vi "State Machine.vi"() -> ()   [LabVIEW 2022 SP3]
uses:
  <vilib>/ErrorRing/Error Ring.xnode
  Control 9.ctl
panel:
  out "value voltage":dbl caption="Current Value (V)"
  out "Low Battery 4":bool caption="Low"
  out "timed out?\nSignal potentiometer":bool caption="Timeout"
  out "Low Battery 3":bool caption="Low"
  out "timed out?\nBattery potentiometer":bool caption="Timeout"
  in  "Knob 2":cluster{dbl, dbl}(knob)={0.0, 30.0} caption="Voltage Threshold" scale=0.0..12.0
  out "Low Battery 2":bool caption="Low"
  out "timed out?\nLink Quality\nThermometer":bool caption="Timeout"
  out "Low Battery":bool caption="Low"
  out "timed out?\nBattery Thermometer":bool caption="Timeout"
  out "Time Stamp 2":timestamp format="%<%d/%m/%y>T"
  out "Time Stamp":timestamp format="%<%H:%M>T"
  in  "Start/ pause":bool
  in  "Stop button":bool
  in  "Knob":cluster{dbl, dbl}(knob)={0.0, 30.0} caption="Temperature Threshold" scale=-20.0..60.0
  out "Meter":dbl(knob) caption="Voltage" scale=0.0..10.0
  out "Thermometer":dbl(slide) caption="Temperature" scale=0.0..100.0
  in  "Error In":errorcluster
  in  "Set lower voltage threshold":sgl=-1.0
  in  "Set upper voltage threshold":sgl=12.0
  out "Too High Voltage":bool
  in  "Set upper temperature threshold":sgl=30.0
  in  "Set lower temperature threshold":sgl=10.0
  out "Too hot":bool
  out "Too cold":bool
  out "min volt":sgl caption="Minimum (V)"
  out "max volt":sgl caption="Maximum (V)"
  out "mean volt":T1 caption="Mean (V)"
  out "min temp":sgl caption="Minimum (°C)"
  out "max temp":sgl caption="Maximum (°C)"
  out "mean temp":sgl caption="Mean (°C)"
  out "temperature":sgl(graph)
  out "voltage":sgl(graph)
  out "Battery Voltage":sgl
  out "Signal > 75 % 2":bool
  out "Signal > 50 % 2":bool
  out "Signal > 25% 2":bool
  out "Signal > 0% 2":bool
  out "Battery > 75 % 2":bool
  out "Battery > 50 % 2":bool
  out "Battery > 25% 2":bool
  out "Battery > 0% 2":bool
  out "Signal > 75 %":bool
  out "Signal > 50 %":bool
  out "Signal > 25%":bool
  out "Signal > 0%":bool
  out "Battery > 75 %":bool
  out "Battery > 50 %":bool
  out "Battery > 25%":bool
  out "Battery > 0%":bool
  out "Low radio signal\nfor potentiometer":errorcluster
  out "Low Battery\nfor potentiometer":errorcluster
  out "No Signal \non thermometer":errorcluster
  out "No Signal\non potentiometer":errorcluster
  out "Low radio signal\nfor thermometer":errorcluster
  out "Low Battery\nfor thermometer":errorcluster
  out "Too Low Voltage":bool
  # "Thermometer"
  # "Potentiometer"
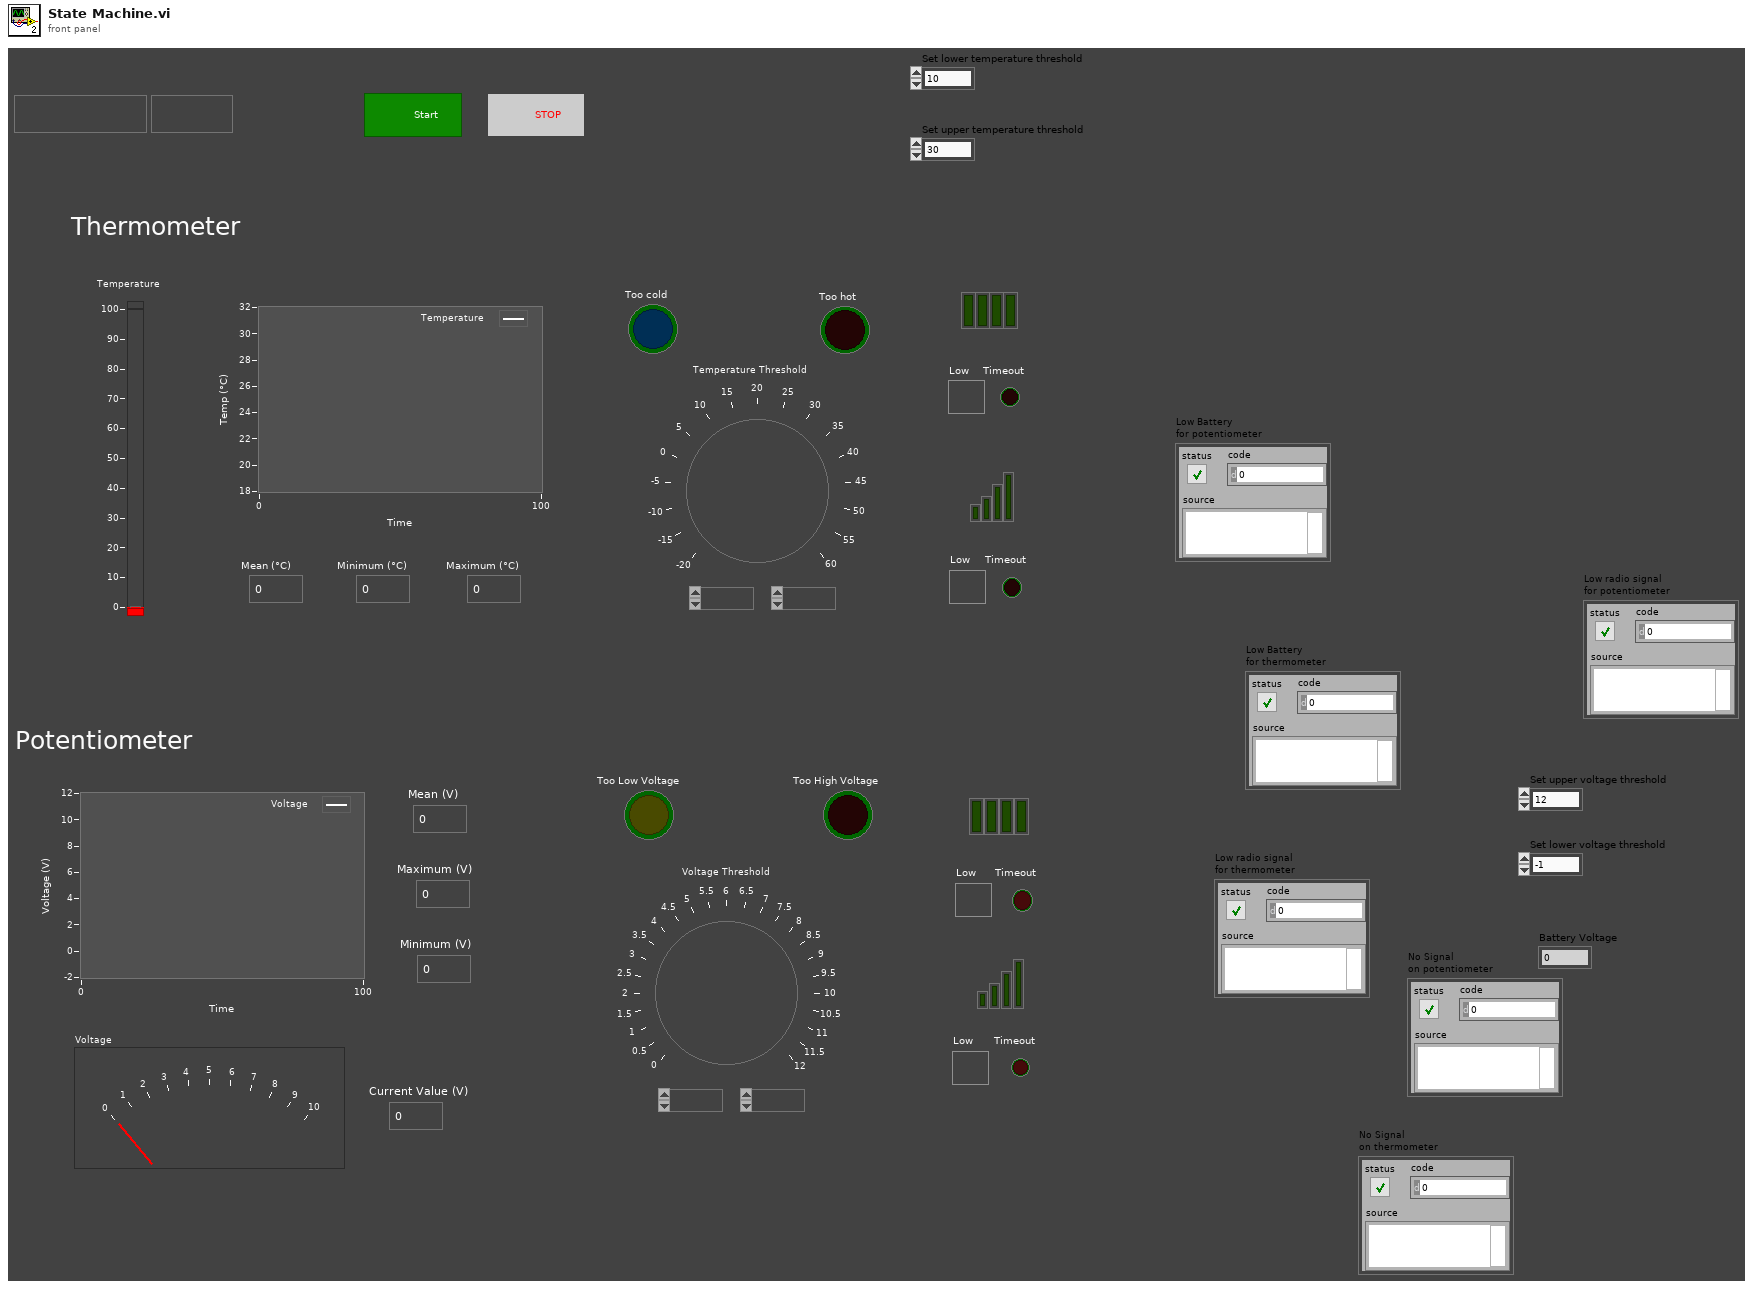
[diagram p1: front panel]
types:
  T1 = typedef "Control 9.ctl" = sgl
  T2 = enum16{"open", "replace", "create", "open or create", "replace or create", "replace or create with confirmation"}
  T3 = enum8{"Enabled", "Disabled", "Disabled and Grayed Out"}
  T4 = enum16{"Error and Alert handler", "Acquisition, calculations and save"}
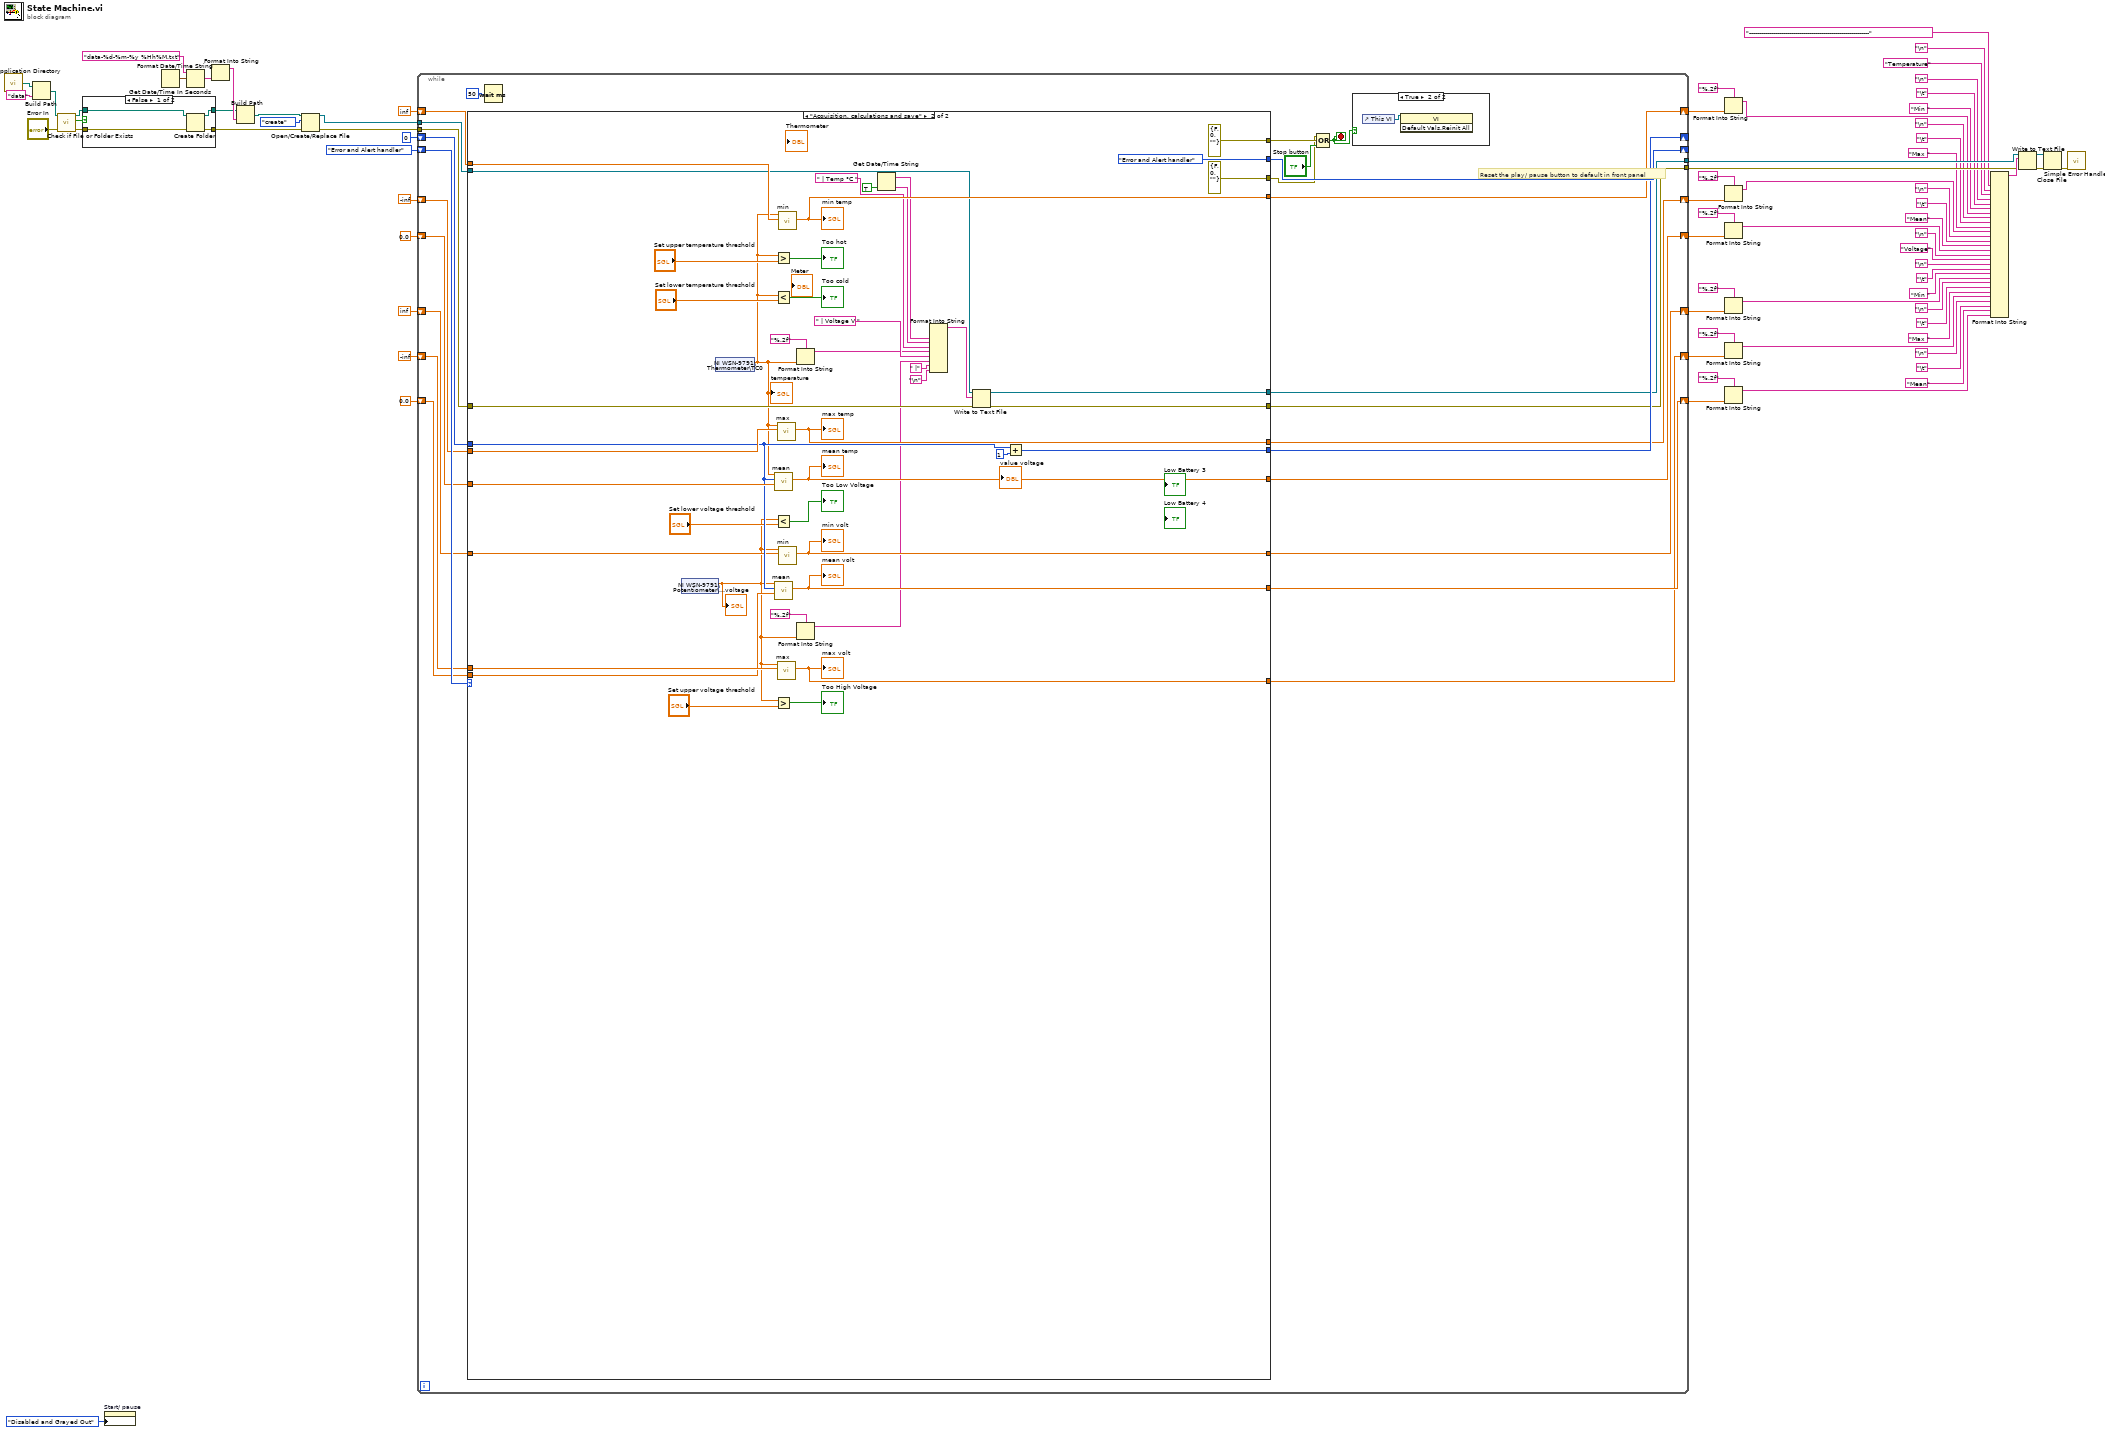
[diagram p0: block diagram]
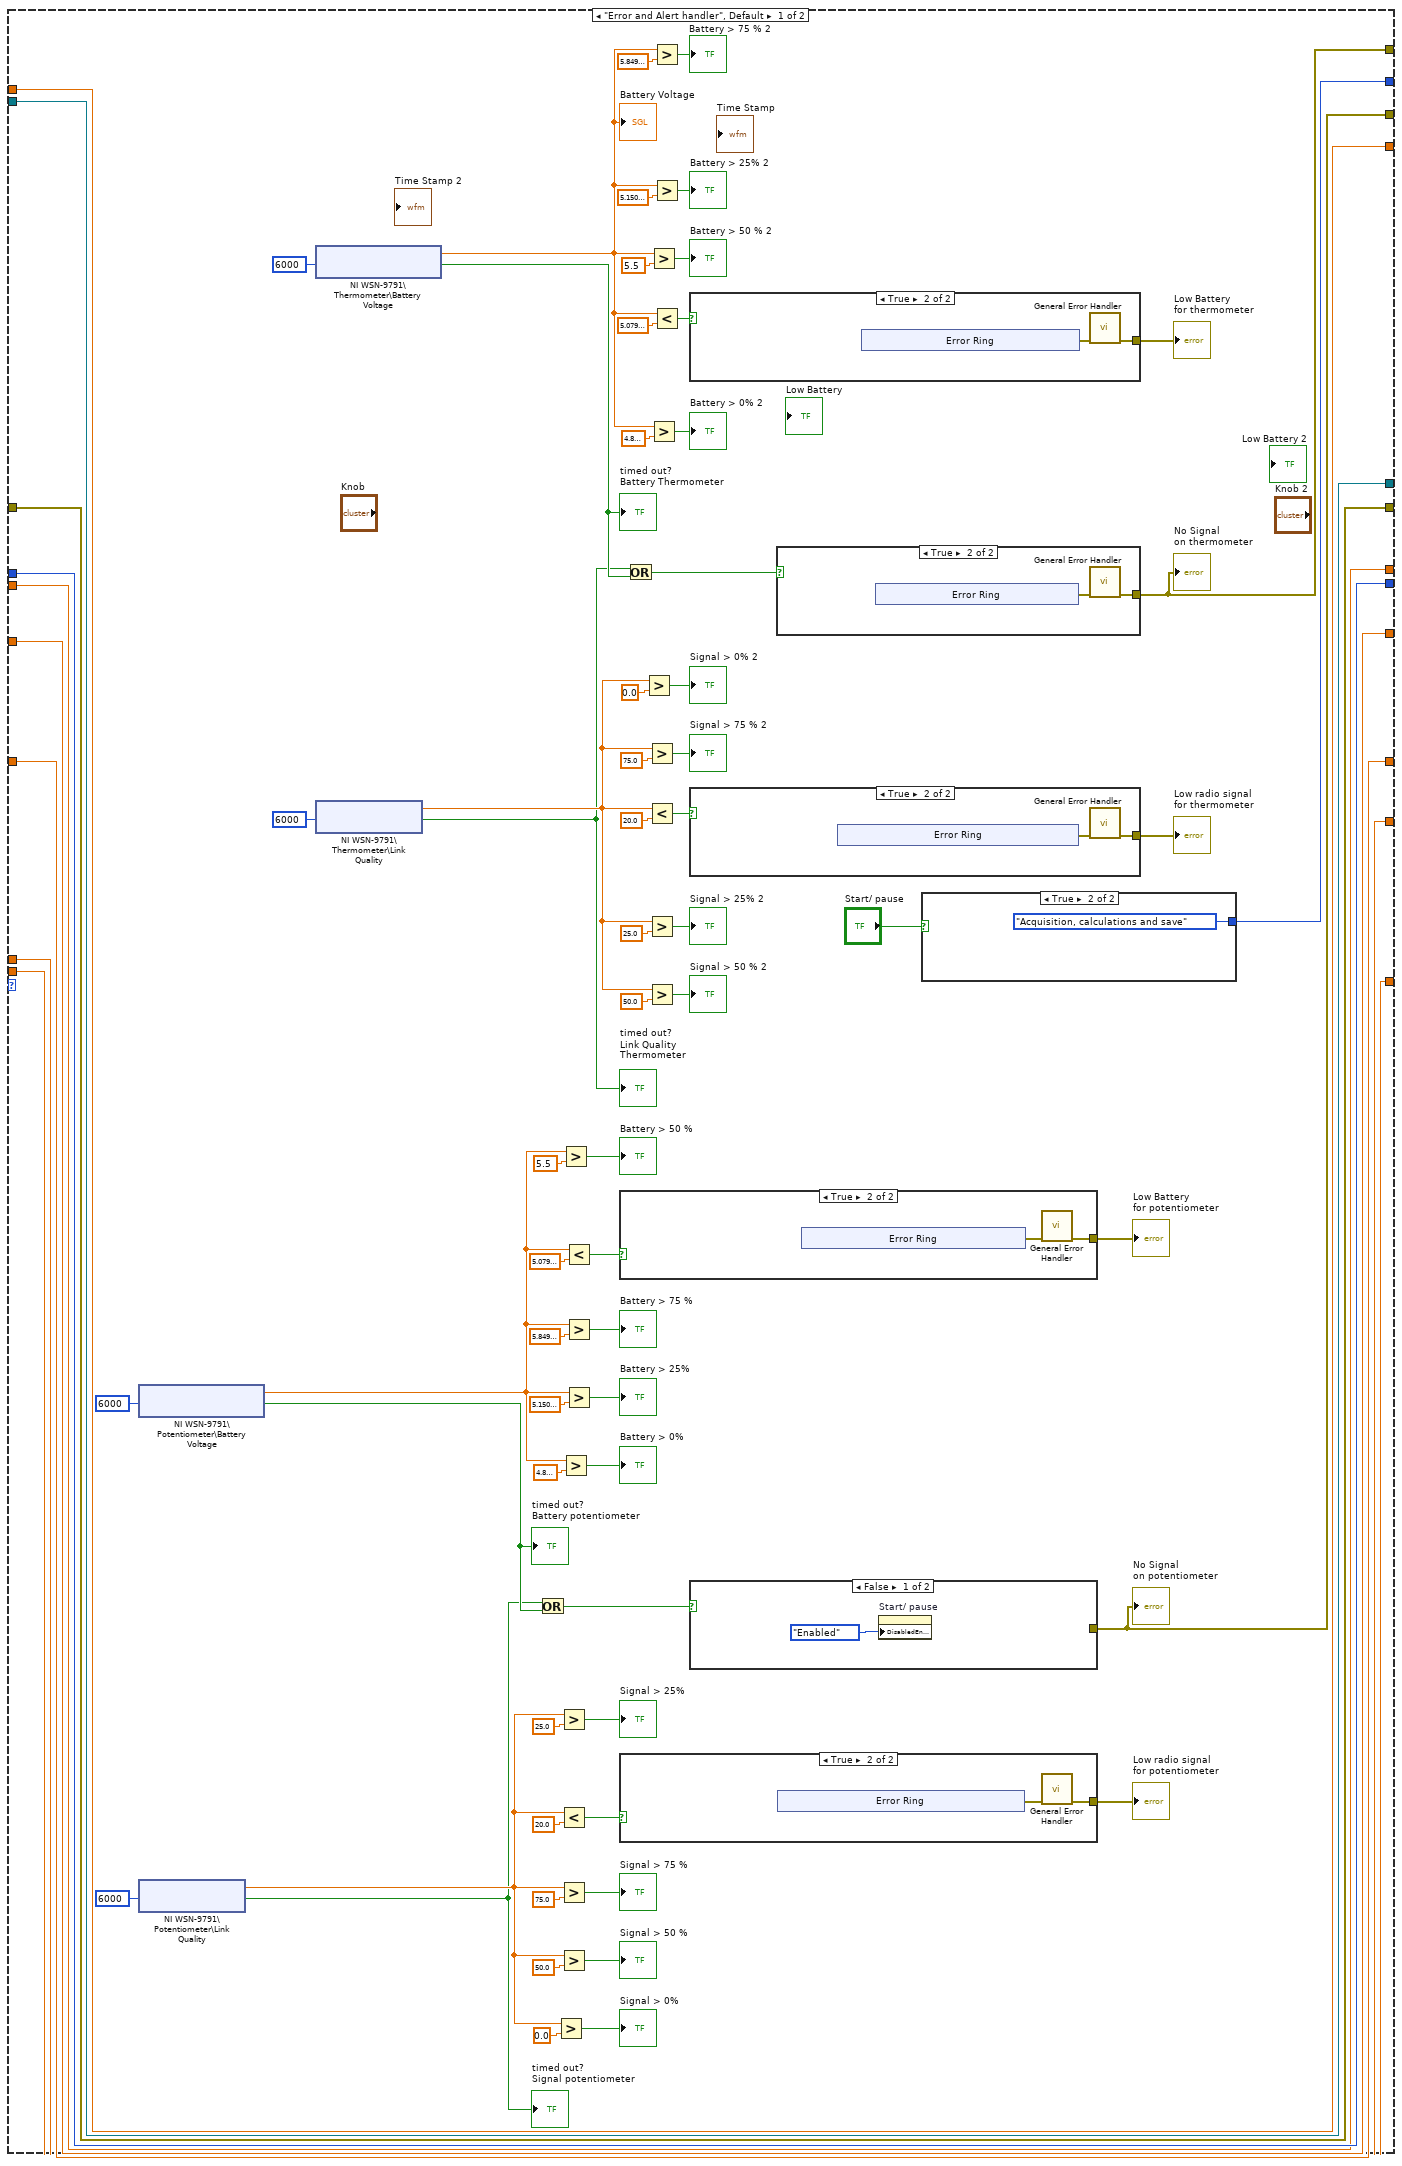
[diagram p4: hidden frame]
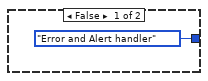
[diagram p5: hidden frame]
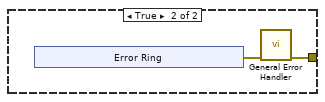
[diagram p9: hidden frame]
diagram:
  n1 = call <vilib>:"Application Directory.vi"() -> ("Application Directory"=w11:path)
  n2 = Build Path(base path=w11, name or relative path="data") -> (appended path=w7:path)
  n3 = call <vilib>:"Check if File or Folder Exists.vi"("error in (no error)"="Error In", "path"=w7) -> ("error out"=w5:errorcluster, "file or folder exists?"=w6:bool, "dup path"=w3:path)  [unwired: 7 in]
  n4 = case shown="False" w6 {
    tunnel: w5 -> [w77 w78]
    tunnel: [w76 w78] -> w4
    tunnel: w3 -> [w75 w79]
    tunnel: [w74 w79] -> w2
    frame False {
      n5 = Create Folder(path (use dialog)=w75, error in=w77) -> (created path=w74:path, error out=w76:errorcluster)  [unwired: 1 in, 1 out]
    }
    frame True {
    }
  }
  n6 = property on="Start/ pause" class="Bool (strict)"("DisabledEnum"=T3."Disabled and Grayed Out" ("Disabled")) -> ()  [unwired: 2 in, 2 out]
  n7 = Get Date/Time In Seconds() -> (seconds since 1Jan1904=w14:timestamp)
  n8 = Format Date/Time String(time format string (%c)="data-%d-%m-%y %Hh%M.txt", seconds (now)=w14) -> (date/time string=w12:string)  [unwired: 1 in]
  n9 = Format Into String(w12) -> (resulting string=w9:string)  [unwired: 3 in, 1 out]
  n10 = Build Path(base path=w2, name or relative path=w9) -> (appended path=w8:path)
  n11 = Open/Create/Replace File(file path (use dialog)=w8, error in=w4, operation (0:open)=T2."create") -> (refnum out=w59:refnum<file>, error out=w56:errorcluster)  [unwired: 3 in, 1 out]
  n12 = while {
    shift-right: [w103] -> _
    shift-left: T4."Error and Alert handler" -> [w99]
    shift-right: [w97] -> _
    shift-left: 0 -> [w98]
    shift-right: [w95] -> w36
    shift-left: sgl 0.0 -> [w96]
    shift-right: [w93] -> w35
    shift-left: -inf -> [w94]
    shift-right: [w91] -> w43
    shift-left: inf -> [w92]
    shift-right: [w87] -> w15
    shift-left: sgl 0.0 -> [w88]
    shift-right: [w86] -> w16
    shift-left: -inf -> [w89]
    shift-right: [w85] -> w17
    shift-left: inf -> [w90]
    tunnel: w59 -> [w83]
    tunnel: [w82] -> w58
    tunnel: [w81] -> w57
    tunnel: w56 -> [w80]
    stop <- w84 stop-if-true
    # "Reset the play/ pause button to default in front panel"
    n13 = case shown="\"Acquisition, calculations and save\"" w99 {
      tunnel: [w108 T4."Error and Alert handler"] -> w103
      tunnel: [w122 errorcluster {"status"=FALSE, "code"=0, "source"=""} ("error out")] -> w101
      tunnel: [w121 errorcluster {"status"=FALSE, "code"=0, "source"=""} ("error out")] -> w100
      tunnel: w98 -> [w116 w228]
      tunnel: [w116 w226] -> w97
      tunnel: w96 -> [w115 w238]
      tunnel: [w115 w237] -> w95
      tunnel: w94 -> [w114 w236]
      tunnel: [w114 w234] -> w93
      tunnel: w92 -> [w113 w235]
      tunnel: [w113 w233] -> w91
      tunnel: w90 -> [w110 w225]
      tunnel: w89 -> [w111 w232]
      tunnel: w88 -> [w112 w231]
      tunnel: [w112 w230] -> w87
      tunnel: [w111 w229] -> w86
      tunnel: [w110 w224] -> w85
      tunnel: w83 -> [w107 w215]
      tunnel: [w107 w214] -> w82
      tunnel: [w106 w213] -> w81
      tunnel: w80 -> [w106 w212]
      frame "Error and Alert handler", Default {
        n14 = shared-variable "NI WSN-9791\\Potentiometer\\Battery Voltage"(6000 ("ms timeout (0)")) -> (w126:sgl, w118:bool)  [unwired: 1 in, 1 out]
        "timed out?\nBattery potentiometer" <- w118
        n15 = shared-variable "NI WSN-9791\\Potentiometer\\Link Quality"(6000 ("ms timeout (0)")) -> (w125:sgl, w117:bool)  [unwired: 1 in, 1 out]
        "timed out?\nSignal potentiometer" <- w117
        n16 = shared-variable "NI WSN-9791\\Thermometer\\Battery Voltage"(6000 ("ms timeout (0)")) -> (w123:sgl, w120:bool)  [unwired: 1 in, 1 out]
        "timed out?\nBattery Thermometer" <- w120
        "Battery Voltage" <- w123
        n17 = shared-variable "NI WSN-9791\\Thermometer\\Link Quality"(6000 ("ms timeout (0)")) -> (w124:sgl, w119:bool)  [unwired: 1 in, 1 out]
        "timed out?\nLink Quality\nThermometer" <- w119
        n18 = Or(x=w117, y=w118) -> (x .or. y?=w174:bool)
        n19 = Greater?(x=w125, y=sgl 0.0) -> (0:→"Signal > 0%":bool)
        n20 = Greater?(x=w125, y=sgl 25.0) -> (0:→"Signal > 25%":bool)
        n21 = Less?(x=w125, y=sgl 20.0) -> (x < y?=w149:bool)
        n22 = Greater?(x=w125, y=sgl 75.0) -> (0:→"Signal > 75 %":bool)
        n23 = Greater?(x=w125, y=sgl 50.0) -> (0:→"Signal > 50 %":bool)
        n24 = Greater?(x=w126, y=sgl 5.5) -> (0:→"Battery > 50 %":bool)
        n25 = Greater?(x=w126, y=sgl 4.8) -> (0:→"Battery > 0%":bool)
        n26 = Less?(x=w126, y=sgl 5.08) -> (x < y?=w168:bool)
        n27 = Greater?(x=w126, y=sgl 5.85) -> (0:→"Battery > 75 %":bool)
        n28 = Greater?(x=w126, y=sgl 5.15) -> (0:→"Battery > 25%":bool)
        n29 = case shown="True" w168 {
          tunnel: [_ w183] -> w172
          frame False {
          }
          frame True {
            n30 = xnode "Error Ring"() -> ("error out"=w182:errorcluster)
            n31 = call <vilib>:"General Error Handler.vi"("error in (no error)"=w182) -> ("error out"=w183:errorcluster)  [unwired: 10 in, 4 out]
          }
        }
        "Low Battery\nfor potentiometer" <- w172
        n32 = case shown="True" w149 {
          tunnel: [_ w180] -> w171
          frame False {
          }
          frame True {
            n33 = xnode "Error Ring"() -> ("error out"=w179:errorcluster)
            n34 = call <vilib>:"General Error Handler.vi"("error in (no error)"=w179) -> ("error out"=w180:errorcluster)  [unwired: 10 in, 4 out]
          }
        }
        "Low radio signal\nfor potentiometer" <- w171
        n35 = Or(x=w119, y=w120) -> (x .or. y?=w173:bool)
        n36 = Greater?(x=w124, y=sgl 0.0) -> (0:→"Signal > 0% 2":bool)
        n37 = Greater?(x=w124, y=sgl 75.0) -> (0:→"Signal > 75 % 2":bool)
        n38 = Less?(x=w124, y=sgl 20.0) -> (x < y?=w130:bool)
        n39 = Greater?(x=w124, y=sgl 25.0) -> (0:→"Signal > 25% 2":bool)
        n40 = Greater?(x=w124, y=sgl 50.0) -> (0:→"Signal > 50 % 2":bool)
        n41 = Greater?(x=w123, y=sgl 5.5) -> (0:→"Battery > 50 % 2":bool)
        n42 = Greater?(x=w123, y=sgl 4.8) -> (0:→"Battery > 0% 2":bool)
        n43 = Greater?(x=w123, y=sgl 5.85) -> (0:→"Battery > 75 % 2":bool)
        n44 = Greater?(x=w123, y=sgl 5.15) -> (0:→"Battery > 25% 2":bool)
        n45 = Less?(x=w123, y=sgl 5.08) -> (x < y?=w127:bool)
        n46 = case shown="True" w127 {
          tunnel: [_ w196] -> w176
          frame False {
          }
          frame True {
            n47 = xnode "Error Ring"() -> ("error out"=w195:errorcluster)
            n48 = call <vilib>:"General Error Handler.vi"("error in (no error)"=w195) -> ("error out"=w196:errorcluster)  [unwired: 10 in, 4 out]
          }
        }
        "Low Battery\nfor thermometer" <- w176
        n49 = case shown="True" w130 {
          tunnel: [_ w193] -> w175
          frame False {
          }
          frame True {
            n50 = xnode "Error Ring"() -> ("error out"=w192:errorcluster)
            n51 = call <vilib>:"General Error Handler.vi"("error in (no error)"=w192) -> ("error out"=w193:errorcluster)  [unwired: 10 in, 4 out]
          }
        }
        "Low radio signal\nfor thermometer" <- w175
        n52 = case shown="False" w174 {
          tunnel: [_ w190] -> w121
          frame False {
            n53 = property on="Start/ pause" class="Bool (strict)"("DisabledEnum"=T3."Enabled" ("Disabled")) -> ()  [unwired: 2 in, 2 out]
          }
          frame True {
            n54 = xnode "Error Ring"() -> ("error out"=w189:errorcluster)
            n55 = call <vilib>:"General Error Handler.vi"("error in (no error)"=w189) -> ("error out"=w190:errorcluster)  [unwired: 10 in, 4 out]
          }
        }
        "No Signal\non potentiometer" <- w121
        n56 = case shown="True" w173 {
          tunnel: [_ w186] -> w122
          frame False {
          }
          frame True {
            n57 = xnode "Error Ring"() -> ("error out"=w185:errorcluster)
            n58 = call <vilib>:"General Error Handler.vi"("error in (no error)"=w185) -> ("error out"=w186:errorcluster)  [unwired: 10 in, 4 out]
          }
        }
        "No Signal \non thermometer" <- w122
        n59 = case shown="True" "Start/ pause" {
          tunnel: [T4."Error and Alert handler" T4."Acquisition, calculations and save"] -> w108
          frame False {
          }
          frame True {
          }
        }
      }
      frame "Acquisition, calculations and save" {
        n60 = shared-variable "NI WSN-9791\\Potentiometer\\AI0"() -> (w203:sgl)  [unwired: 1 in, 1 out]
        "voltage" <- w203
        n61 = shared-variable "NI WSN-9791\\Thermometer\\TC0"() -> (w198:sgl)  [unwired: 1 in, 1 out]
        "temperature" <- w198
        n62 = Greater?(x=w198, y="Set upper temperature threshold") -> (0:→"Too hot":bool)
        n63 = Less?(x=w198, y="Set lower temperature threshold") -> (x < y?=→"Too cold":bool)
        n64 = call "mean.vi"("Numeric 2"=w238, "n"=w228, "Numeric"=w198) -> ("mean"=w237:sgl)  [unwired: 8 in]
        "mean temp" <- w237
        n65 = Less?(x=w203, y="Set lower voltage threshold") -> (x < y?=→"Too Low Voltage":bool)
        n66 = call "mean.vi"("Numeric 2"=w231, "n"=w228, "Numeric"=w203) -> ("mean"=w230:sgl)  [unwired: 8 in]
        "mean volt" <- w230
        n67 = Greater?(x=w203, y="Set upper voltage threshold") -> (0:→"Too High Voltage":bool)
        n68 = call "max.vi"("Numeric 3"=w236, "Numeric in"=w198) -> ("max"=w234:sgl)  [unwired: 9 in]
        "max temp" <- w234
        n69 = call "max.vi"("Numeric 3"=w232, "Numeric in"=w203) -> ("max"=w229:sgl)  [unwired: 9 in]
        "max volt" <- w229
        n70 = call "min.vi"("Numeric"=w235, "Numeric 2"=w198) -> ("min"=w233:sgl)  [unwired: 9 in]
        "min temp" <- w233
        n71 = call "min.vi"("Numeric"=w225, "Numeric 2"=w203) -> ("min"=w224:sgl)  [unwired: 9 in]
        "min volt" <- w224
        n72 = Format Into String(format string="%.2f", w198) -> (resulting string=w199:string)  [unwired: 2 in, 1 out]
        n73 = Format Into String(format string="%.2f", w203) -> (resulting string=w201:string)  [unwired: 2 in, 1 out]
        n74 = Get Date/Time String(want seconds? (F)=TRUE) -> (date string=w210:string, time string=w209:string)  [unwired: 2 in]
        n75 = Format Into String(w210, w209, " | Temp °C " ("input 3"), w199, " | Voltage V " ("input 5"), w201, " |" ("input 7"), "\n") -> (resulting string=w211:string)  [unwired: 3 in, 1 out]
        n76 = Write to Text File(file (use dialog)=w215, text=w211, error in=w212) -> (refnum out=w214:refnum<file>, error out=w213:errorcluster)  [unwired: 1 in, 1 out]
        n77 = Add(x=w228, y=1) -> (x+y=w226:i32)
      }
    }
    n78 = Wait (ms)(milliseconds to wait=u32 50) -> ()  [unwired: 1 out]
    n79 = Compound Arithmetic op=OR(w100, w101, "Stop button") -> (w84:bool)
    n80 = case shown="True" w84 {
      frame False {
      }
      frame True {
        n81 = control-ref of="This VI"() -> (w105:refnum<vi>)
        n82 = invoke class="VI" method="Default Vals.Reinit All"(reference=w105) -> ()  [unwired: 2 in, 3 out]
      }
    }
  }
  n83 = Format Into String(format string="%.2f", w43) -> (resulting string=w41:string)  [unwired: 2 in, 1 out]
  n84 = Format Into String(format string="%.2f", w35) -> (resulting string=w39:string)  [unwired: 2 in, 1 out]
  n85 = Format Into String(format string="%.2f", w36) -> (resulting string=w37:string)  [unwired: 2 in, 1 out]
  n86 = Format Into String(format string="%.2f", w17) -> (resulting string=w28:string)  [unwired: 2 in, 1 out]
  n87 = Format Into String(format string="%.2f", w16) -> (resulting string=w23:string)  [unwired: 2 in, 1 out]
  n88 = Format Into String(format string="%.2f", w15) -> (resulting string=w18:string)  [unwired: 2 in, 1 out]
  n89 = Format Into String("------------------------------------------------------------" ("input 1"), "\n", "Temperature" ("input 1"), "\n", "\t", "Min " ("input 1"), w41, "\n", "\t", "Max " ("input 1"), w39, "\n", "\t", "Mean" ("input 1"), w37, "\n", "Voltage" ("input 1"), "\n", "\t", "Min " ("input 1"), w28, "\n", "\t", "Max " ("input 1"), w23, "\n", "\t", "Mean" ("input 1"), w18) -> (resulting string=w60:string)  [unwired: 3 in, 1 out]
  n90 = Write to Text File(file (use dialog)=w58, text=w60, error in=w57) -> (refnum out=w62:refnum<file>, error out=w61:errorcluster)  [unwired: 1 in, 1 out]
  n91 = Close File(refnum=w62, error in=w61) -> (error out=w63:errorcluster)  [unwired: 1 out]
  n92 = call <vilib>:"Simple Error Handler.vi"("error in (no error)"=w63) -> ()  [unwired: 4 in, 5 out]
